vi "Get Instrument Type ID.vi"(8 "error in":errorcluster, 11 "session factory in":refnum<class "Abstract_Instrument.lvclass">) -> (0 "error out":errorcluster, 2 "instrument type id":string, 3 "session factory out":refnum<class "Abstract_Instrument.lvclass">)   [LabVIEW 2021, in "Abstract_Instrument.lvclass"]
doc: "Returns the type ID for the instrument in the pin map file. When using third party instruments not natively supported by the pin map editor, you must create a custom instrument in the pin map file and assign it a unique instrument type ID. Return the same instrument type ID from this method to access the third party instrument from within MeasurementLink."
uses:
  Abstract_Instrument.lvclass
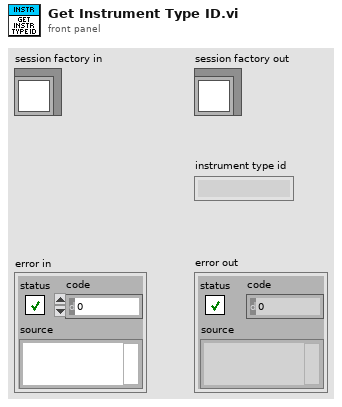
[diagram p1: front panel]
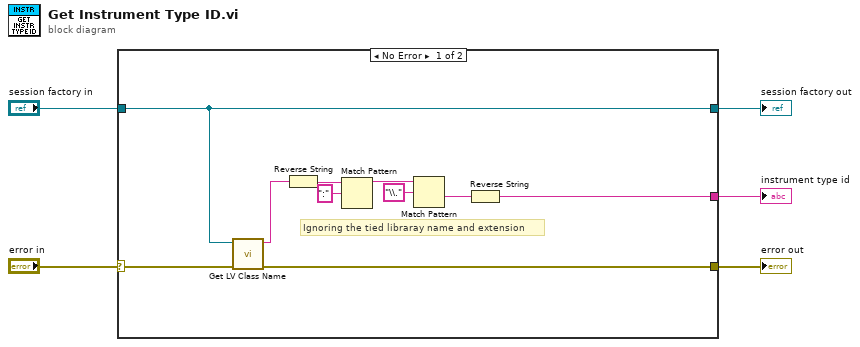
[diagram p0: block diagram]
diagram:
  n1 = case shown="No Error" "error in" {
    selector: "error in" -> [w8 w17]
    tunnel: [w7 w17] -> w2
    tunnel: [w9 w16] -> w4
    tunnel: "session factory in" -> [w9 w16]
    tunnel: [w6 _] -> w1
    frame No Error {
      # "Ignoring the tied libraray name and extension"
      n2 = call <vilib>:"Get LV Class Name.vi"("error in (no error)"=w8, "object"=w9) -> ("error out"=w7:errorcluster, "class name"=w15:string)  [unwired: 8 in]
      n3 = Reverse String(1:w15) -> (0:w14:string)
      n4 = Match Pattern(string=w14, regular expression=":") -> (before substring=w12:string)  [unwired: 1 in, 3 out]
      n5 = Match Pattern(string=w12, regular expression="\\.") -> (after substring=w10:string)  [unwired: 1 in, 3 out]
      n6 = Reverse String(1:w10) -> (0:w6:string)
    }
    frame Error {
    }
  }
  "error out" <- w2
  "session factory out" <- w4
  "instrument type id" <- w1
